vi "First.vi"(0 "object in":refnum<class "Iterator.lvclass">, 5 "Error In":errorcluster) -> (14 "object out":refnum<class "Iterator.lvclass">, 16 "Root":refnum<class "Node.lvclass">, 19 "Error Out":errorcluster)   [LabVIEW 2024, in "Iterator.lvclass"]
doc: "Returns root of the collection"
uses:
  Iterator.lvclass
  Node_class/Node.lvclass
panel:
  # "Connector Pane"
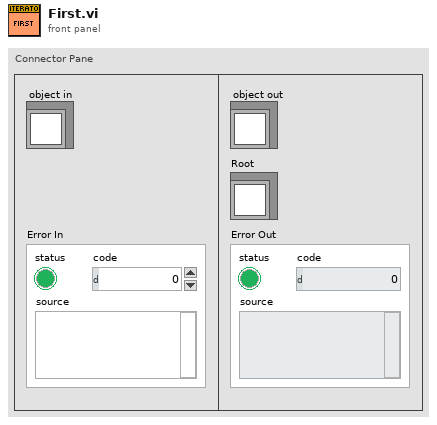
[diagram p1: front panel]
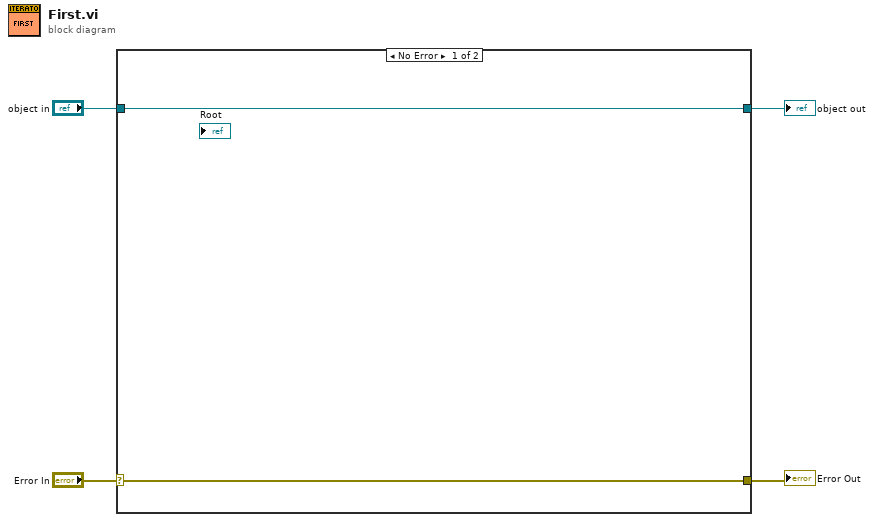
[diagram p0: block diagram]
diagram:
  n1 = case shown="No Error" "Error In" {
    selector: "Error In" -> [w6 w8]
    tunnel: [w6 w8] -> w3
    tunnel: [w5 w7] -> w1
    tunnel: "object in" -> [w5 w7]
    frame No Error {
    }
    frame Error {
    }
  }
  "Error Out" <- w3
  "object out" <- w1
